vi "CfgFile Set Desc c.vi"(8 "error in (no error)":errorcluster, 10 "c":T1, 11 "LF2R IDE in":refnum<class "LF2R IDE.lvclass">) -> (0 "error out":errorcluster, 3 "LF2R IDE out":refnum<class "LF2R IDE.lvclass">)   [LabVIEW 2018, in "LF2R IDE.lvlib" / "LF2R IDE.lvclass"]
uses:
  LF2R IDE.lvclass
  Const UI Desc Frame c.ctl
  Const UI Desc Property.ctl
  LF2R IDE.lvclass/LF2R IDE.ctl
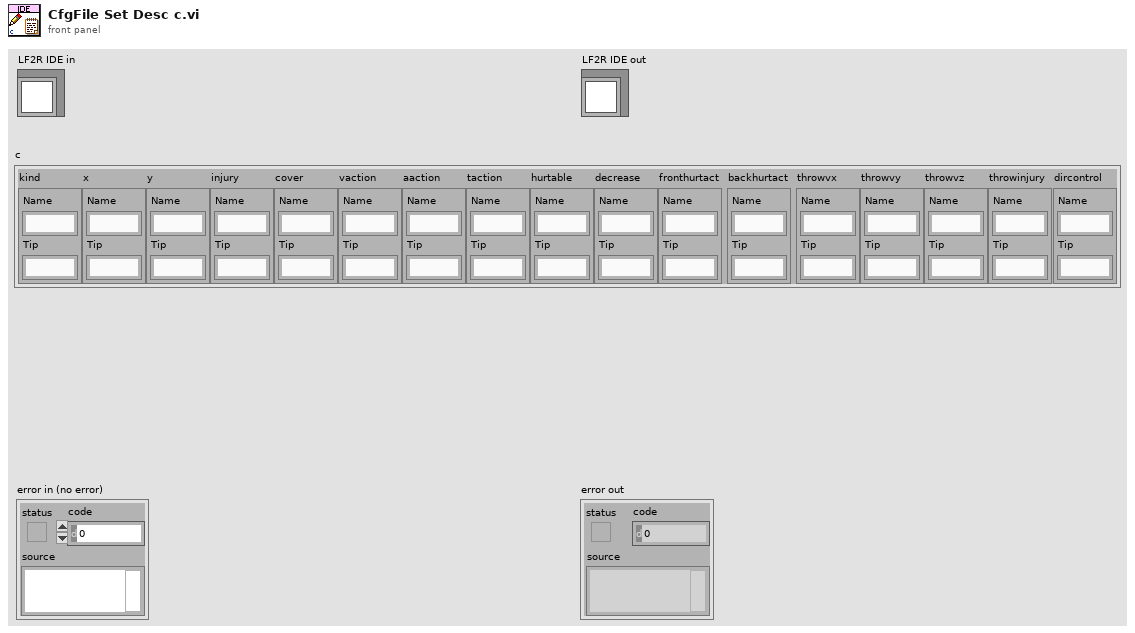
[diagram p1: front panel]
types:
  T1 = typedef "LF2R IDE.lvlib/LF2R IDE.lvclass/Const UI Desc Frame c.ctl" = cluster{"kind":T2, "x":T2, "y":T2, "injury":T2, "cover":T2, "vaction":T2, "aaction":T2, "taction":T2, "hurtable":T2, "decrease":T2, "fronthurtact":T2, "backhurtact":T2, "throwvx":T2, "throwvy":T2, "throwvz":T2, "throwinjury":T2, "dircontrol":T2}
  T2 = typedef "LF2R IDE.lvlib/LF2R IDE.lvclass/Const UI Desc Property.ctl" = cluster{"Name":string, "Tip":string}
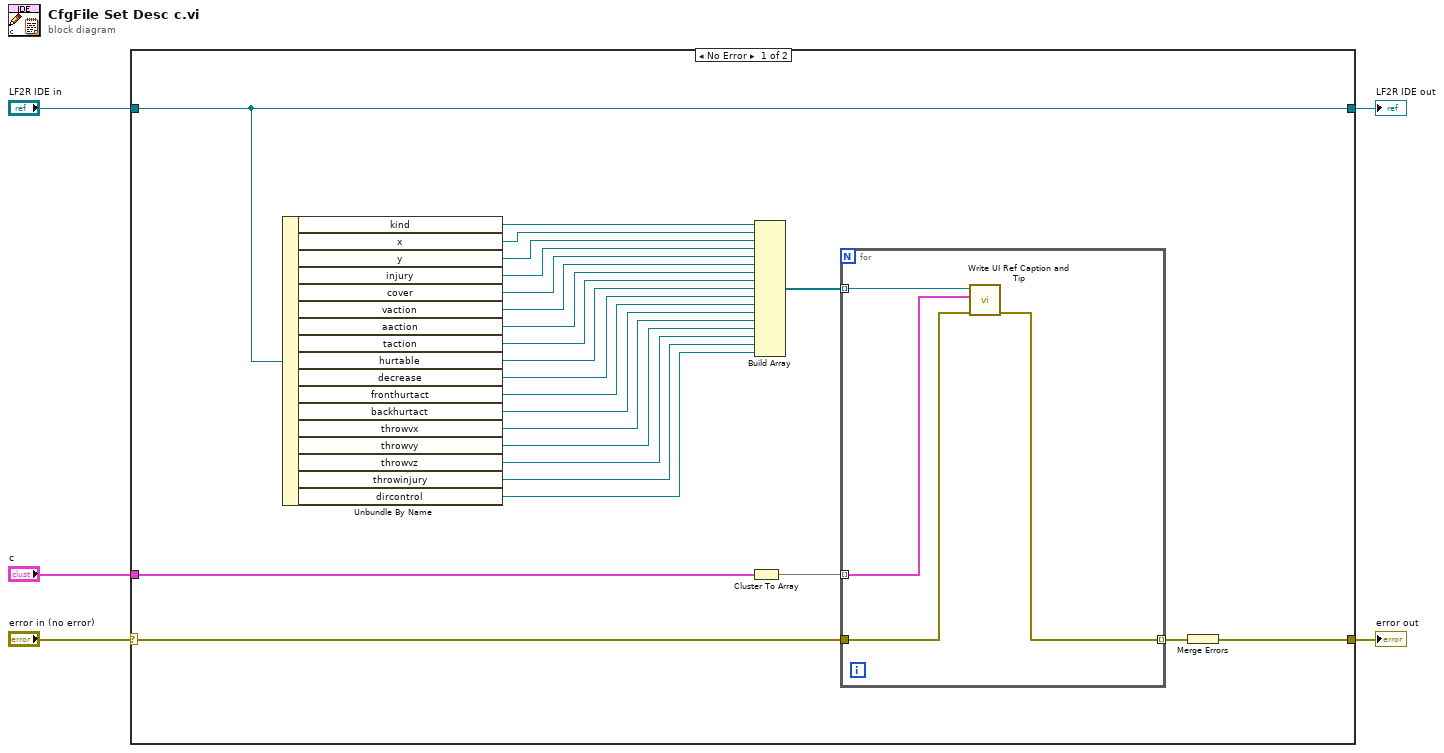
[diagram p0: block diagram]
diagram:
  n1 = case shown="No Error" "error in (no error)" {
    selector: "error in (no error)" -> [w25 w35]
    tunnel: [w23 w35] -> w4
    tunnel: [w29 w34] -> w2
    tunnel: "LF2R IDE in" -> [w29 w34]
    tunnel: "c" -> [w27 _]
    frame No Error {
      n2 = Unbundle By Name(w29) -> ("kind"=w22:refnum<vi>, "x"=w21:refnum<vi>, "y"=w20:refnum<vi>, "injury"=w19:refnum<vi>, "cover"=w18:refnum<vi>, "vaction"=w17:refnum<vi>, "aaction"=w16:refnum<vi>, "taction"=w15:refnum<vi>, "hurtable"=w14:refnum<vi>, "decrease"=w13:refnum<vi>, "fronthurtact"=w12:refnum<vi>, "backhurtact"=w11:refnum<vi>, "throwvx"=w10:refnum<vi>, "throwvy"=w9:refnum<vi>, "throwvz"=w8:refnum<vi>, "throwinjury"=w7:refnum<vi>, "dircontrol"=w6:refnum<vi>)
      n3 = Cluster To Array(cluster=w27) -> (array=w26:T2[])
      n4 = Build Array(w22, w21, w20, w19, w18, w17, w16, w15, w14, w13, w12, w11, w10, w9, w8, w7, w6) -> (w28:refnum<vi>[])
      n5 = for {
        tunnel: w28 -> [w30] mode=indexing
        tunnel: w26 -> [w33] mode=indexing
        tunnel: w25 -> [w32]
        tunnel: [w31] -> w24 mode=indexing
        n6 = call "Write UI Ref Caption and Tip.vi"("error in (no error)"=w32, "UI Property"=w33, "UI Ref"=w30) -> ("error out"=w31:errorcluster)  [unwired: 8 in]
      }
      n7 = Merge Errors(w24) -> (w23:errorcluster)
    }
    frame Error {
    }
  }
  "error out" <- w4
  "LF2R IDE out" <- w2
